vi "Get Recursive File details.vi"(9 "Recursive?":bool, 11 "Path":path) -> (1 "Count":i32, 3 "File Details":path[](array[path]))   [LabVIEW 2010]
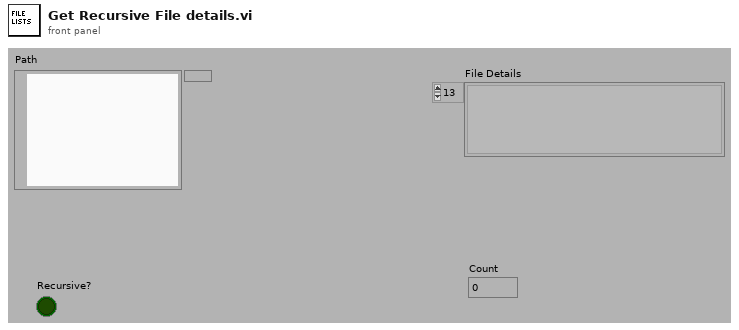
[diagram p1: front panel]
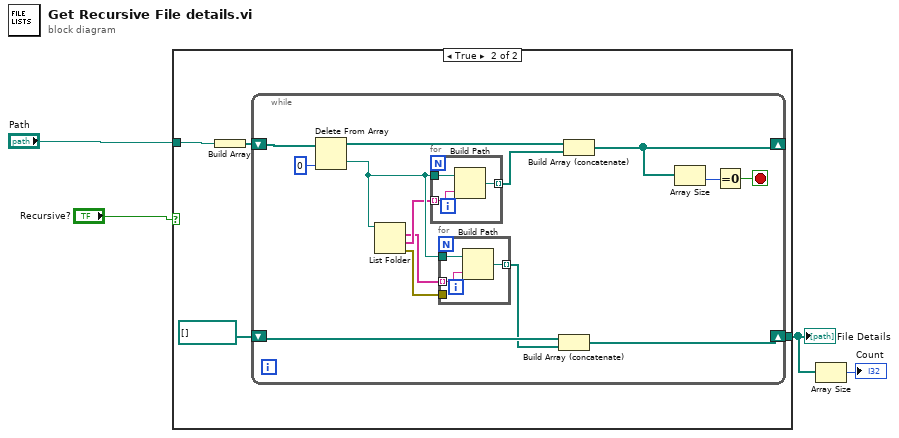
[diagram p0: block diagram]
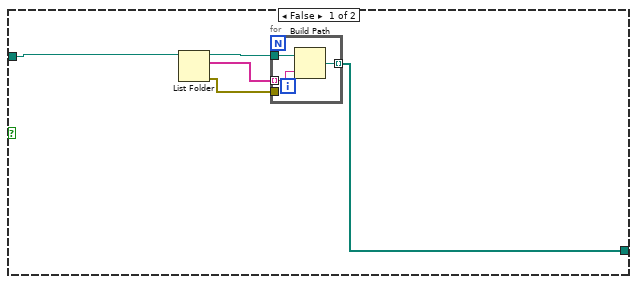
[diagram p2: hidden frame]
diagram:
  n1 = case shown="True" "Recursive?" {
    tunnel: "Path" -> [w8 w15]
    tunnel: [w6 w13] -> w1
    frame False {
      n2 = List Folder(path=w8) -> (path out=w7:path, filenames=w9:string[], error out=w5:errorcluster)  [unwired: 3 in, 1 out]
      n3 = for {
        tunnel: w9 -> [w12] mode=indexing
        tunnel: w7 -> [w11]
        tunnel: [w10] -> w6 mode=indexing
        tunnel: w5 -> [_]
        n4 = Build Path(base path=w11, name or relative path=w12) -> (appended path=w10:path)
      }
    }
    frame True {
      n5 = Build Array(w15) -> (w16:path[])
      n6 = while {
        shift-right: [w19] -> _
        shift-left: w16 -> [w30]
        shift-right: [w20] -> w13
        shift-left: path[] [] ("appended array") -> [w22]
        stop <- w28 stop-if-true
        n7 = Delete From Array(array=w30, index=0) -> (deleted portion=w26:path, array with subset deleted=w24:path[])  [unwired: 1 in]
        n8 = List Folder(path=w26) -> (filenames=w18:string[], folder names=w25:string[], error out=w17:errorcluster)  [unwired: 3 in, 1 out]
        n9 = for {
          tunnel: w25 -> [w36] mode=indexing
          tunnel: w26 -> [w35]
          tunnel: [w34] -> w23 mode=indexing
          n10 = Build Path(base path=w35, name or relative path=w36) -> (appended path=w34:path)
        }
        n11 = for {
          tunnel: w18 -> [w33] mode=indexing
          tunnel: w26 -> [w32]
          tunnel: [w31] -> w21 mode=indexing
          tunnel: w17 -> [_]
          n12 = Build Path(base path=w32, name or relative path=w33) -> (appended path=w31:path)
        }
        n13 = Build Array (concatenate)(w22, w21) -> (w20:path[])
        n14 = Build Array (concatenate)(w24, w23) -> (w19:path[])
        n15 = Array Size(array=w19) -> (size(s)=w27:i32)
        n16 = Equal To 0?(x=w27) -> (x = 0?=w28:bool)
      }
    }
  }
  "File Details" <- w1
  n17 = Array Size(array=w1) -> (size(s)=→"Count":i32)
